vi "Sample Method with Same Control Names.vi"(8 "error in (no error)":errorcluster, 9 "String":string, 10 "Numeric In":dbl, 11 "My Sample Class in":refnum<class "My Sample Class.lvclass">) -> (0 "error out":errorcluster, 1 "Numeric Out":dbl, 2 "Boolean":bool, 3 "My Sample Class out":refnum<class "My Sample Class.lvclass">)   [LabVIEW 2016, in "SLL Scripting.lvlib" / "My Sample Class.lvclass"]
uses:
  My Sample Class.lvclass
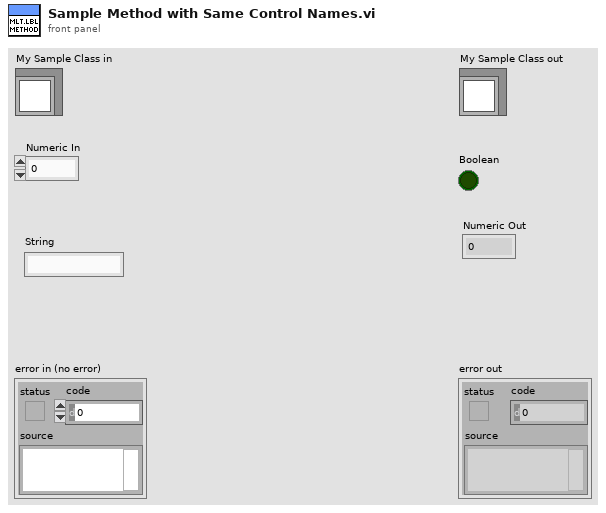
[diagram p1: front panel]
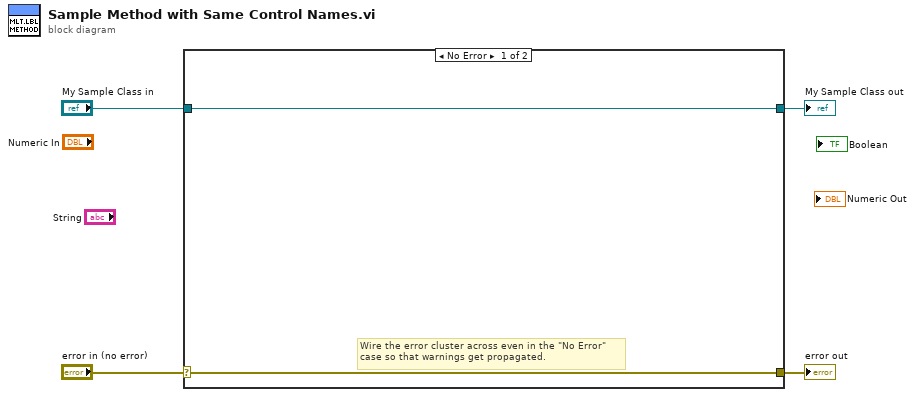
[diagram p0: block diagram]
diagram:
  n1 = case shown="No Error" "error in (no error)" {
    selector: "error in (no error)" -> [w5 w8]
    tunnel: [w5 w8] -> w3
    tunnel: [w6 w7] -> w1
    tunnel: "My Sample Class in" -> [w6 w7]
    frame No Error {
      # "Wire the error cluster across even in the \"No Error\"\ncase so that warnings get propagated."
    }
    frame Error {
    }
  }
  "error out" <- w3
  "My Sample Class out" <- w1
